vi "bats.parser.runHostTests.vi"() -> ()   [LabVIEW 2020]
uses:
  Market.Data.Common/host/fpganow.common.host.lvlib
panel:
  out "Results.out":T1
  out "error out":errorcluster
  in  "error in":errorcluster
  in  "filter(s)":string[](array[string])=["tests"]
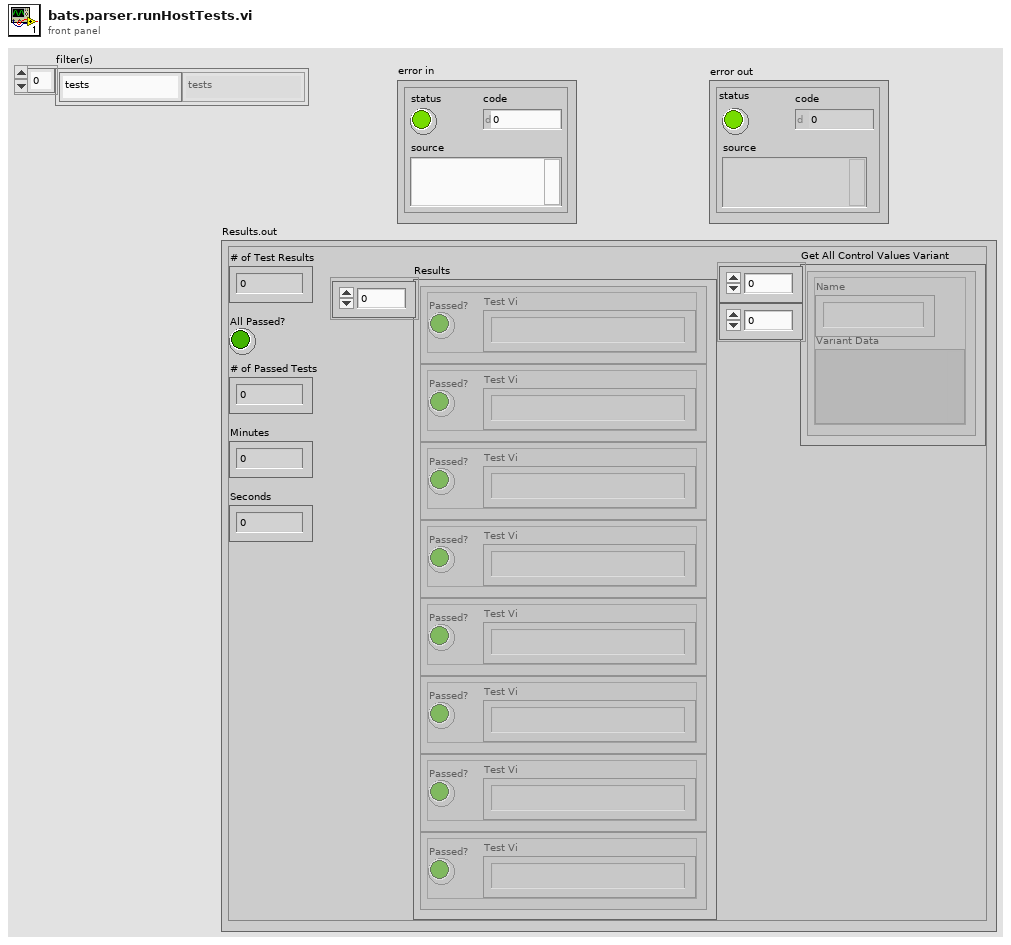
[diagram p1: front panel]
types:
  T1 = cluster{"Results":cluster{"Test Vi":string, "Passed?":bool}[], "# of Test Results":i32, "All Passed?":bool, "# of Passed Tests":i32, "Minutes":u32, "Seconds":u32, "Get All Control Values Variant":cluster{"Name":string, "Variant Data":variant}[][]}
  T2 = cluster{"filter(s)":string[], "path":path, "error in":errorcluster}
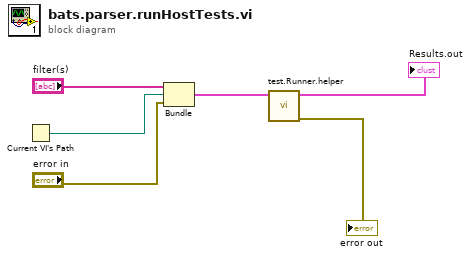
[diagram p0: block diagram]
diagram:
  n1 = Current VI's Path() -> (path=w5:path)
  n2 = Bundle("filter(s)"="filter(s)", "path"=w5, "error in"="error in") -> (w3:T2)  [unwired: 1 in]
  n3 = call "test.Runner.helper.vi"("Parameters.in"=w3) -> ("error out"=→"error out":errorcluster, "Results.out"=→"Results.out":T1)  [unwired: 9 in]
